vi "SERIAL_PROTEUS.vi"() -> ()   [LabVIEW 2020]
uses:
  <vilib>/Instr/_visa.llb/VISA Configure Serial Port (Instr).vi
panel:
  in  "LED 4":bool
  in  "LED 3":bool
  in  "LED 2":bool
  in  "LED 1":bool
  in  "Puerto Serial":refnum<visa-resource-name>
  in  "stop":bool
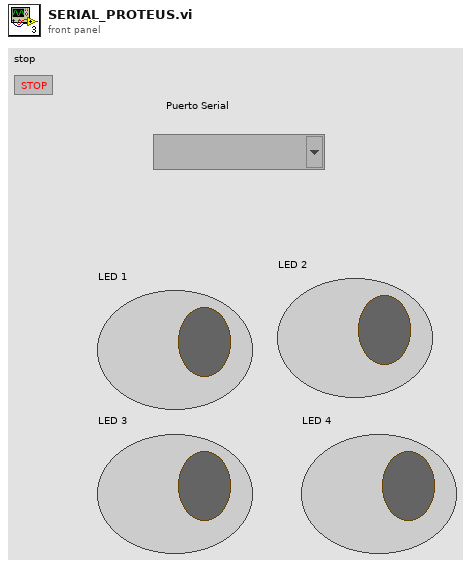
[diagram p1: front panel]
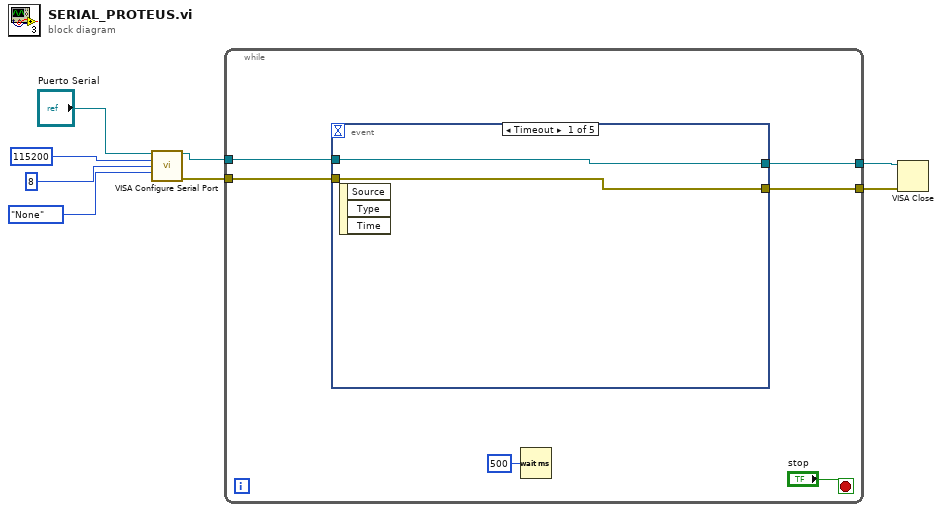
[diagram p0: block diagram]
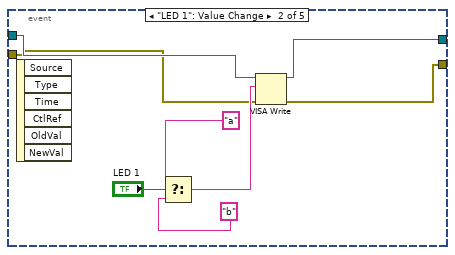
[diagram p2: hidden frame]
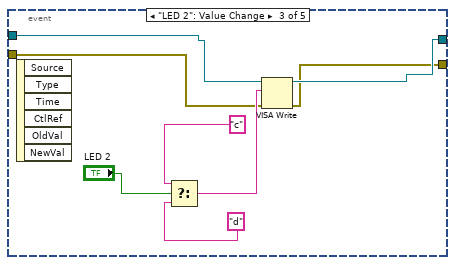
[diagram p3: hidden frame]
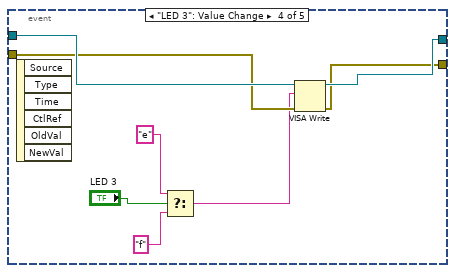
[diagram p4: hidden frame]
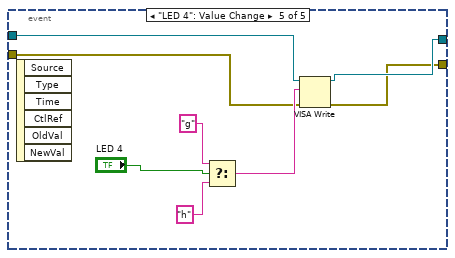
[diagram p5: hidden frame]
diagram:
  n1 = call-poly "VISA Configure Serial Port"("VISA resource name"="Puerto Serial", "baud rate (9600)"=u32 115200, "data bits (8)"=u16 8, "parity (0:none)"=enum16{"None", "Odd", "Even", "Mark", "Space"}."None") -> ("VISA resource name out"=w4:refnum<visa-resource-name>, "error out"=w3:errorcluster)  [unwired: 10 in]
  n2 = while {
    tunnel: w4 -> [w11]
    tunnel: w3 -> [w10]
    tunnel: [w12] -> w2
    tunnel: [w9] -> w1
    stop <- "stop" stop-if-true
    n3 = event shown="[0] Timeout" {
      selector: _ -> [_ _ _ _ _]
      dyn-events: _ -> [_ _ _ _ _]
      timeout: _ -> [_ _ _ _ _]
      tunnel: [w16 w18 w28 w34 w43] -> w12
      tunnel: w11 -> [w16 w20 w26 w37 w45]
      tunnel: w10 -> [w15 w19 w25 w36 w44]
      tunnel: [w15 w17 w27 w33 w42] -> w9
      event Timeout {
        n4 = event-data() -> ()  [unwired: 1 in, 3 out]
      }
      event "LED 1": Value Change {
        n5 = event-data() -> ()  [unwired: 1 in, 6 out]
        n6 = Select(t="a", s="LED 1", f="b") -> (s? t:f=w21:string)
        n7 = VISA Write(VISA resource name=w20, write buffer=w21, error in (no error)=w19) -> (VISA resource name out=w18:refnum<visa-resource-name>, error out=w17:errorcluster)  [unwired: 1 out]
      }
      event "LED 2": Value Change {
        n8 = event-data() -> ()  [unwired: 1 in, 6 out]
        n9 = Select(t="c", s="LED 2", f="d") -> (s? t:f=w32:string)
        n10 = VISA Write(VISA resource name=w26, write buffer=w32, error in (no error)=w25) -> (VISA resource name out=w28:refnum<visa-resource-name>, error out=w27:errorcluster)  [unwired: 1 out]
      }
      event "LED 3": Value Change {
        n11 = event-data() -> ()  [unwired: 1 in, 6 out]
        n12 = Select(t="e", s="LED 3", f="f") -> (s? t:f=w35:string)
        n13 = VISA Write(VISA resource name=w37, write buffer=w35, error in (no error)=w36) -> (VISA resource name out=w34:refnum<visa-resource-name>, error out=w33:errorcluster)  [unwired: 1 out]
      }
      event "LED 4": Value Change {
        n14 = event-data() -> ()  [unwired: 1 in, 6 out]
        n15 = Select(t="g", s="LED 4", f="h") -> (s? t:f=w48:string)
        n16 = VISA Write(VISA resource name=w45, write buffer=w48, error in (no error)=w44) -> (VISA resource name out=w43:refnum<visa-resource-name>, error out=w42:errorcluster)  [unwired: 1 out]
      }
    }
    n17 = Wait (ms)(milliseconds to wait=u32 500) -> ()  [unwired: 1 out]
  }
  n18 = VISA Close(VISA resource name=w2, error in (no error)=w1) -> ()  [unwired: 1 out]
